vi "Delete_unwanted_rows.vi"(1 "Selected Rows":i32[](array[numeric]), 2 "Filename":path) -> ()   [LabVIEW 2015]
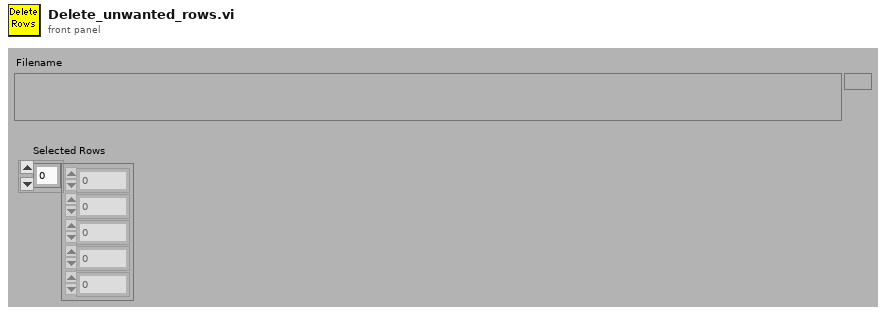
[diagram p1: front panel]
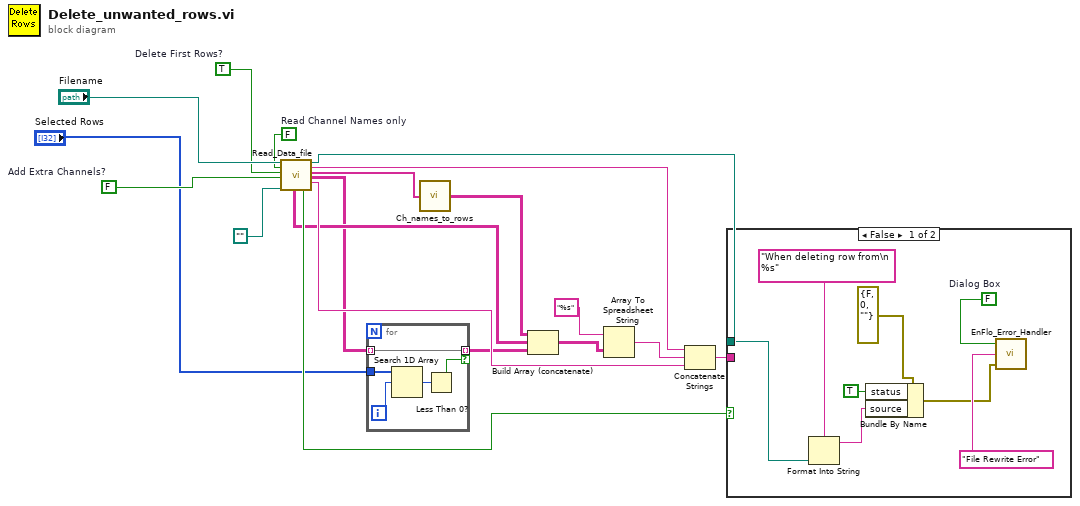
[diagram p0: block diagram]
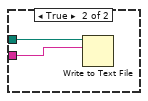
[diagram p2: hidden frame]
diagram:
  w1 = TRUE  # Delete First Rows?
  w5 = FALSE  # Add Extra Channels?
  w17 = FALSE  # Read Channel Names only
  n1 = call "Read_Data_file.vi"("Results file"="Filename", "Read Channel Names only"=w17, "Delete First Rows?"=w1, "Add Extra Channels?"=w5, "Template File"=path "") -> ("Deleted Rows"=w6:string[][], "EOF?"=w7:bool, "Results file Out"=w8:path, "String Before"=w15:string, "Ch names Out"=w14:string[], "Channel Values Out"=w3:string[][], "String After"=w10:string)  [unwired: 1 in, 7 out]
  n2 = for {
    tunnel: "Selected Rows" -> [w24]
    tunnel: w3 -> [w21] mode=indexing
    tunnel: [w21] -> w2 mode=indexing if=w20
    i -> [w23]
    n3 = Search 1D Array(1D array=w24, element=w23) -> (index of element=w22:i32)  [unwired: 1 in]
    n4 = Less Than 0?(x=w22) -> (x < 0?=w20:bool)
  }
  n5 = call "Ch_names_to_rows.vi"("Channel Names"=w14) -> ("3 Row names"=w13:string[][])
  n6 = Build Array (concatenate)(w13, w6, w2) -> (w12:string[][])
  n7 = Array To Spreadsheet String(array=w12, 3:"%s" ("format string")) -> (spreadsheet string=w11:string)  [unwired: 1 in]
  n8 = Concatenate Strings(w15, w11, w10) -> (w9:string)
  n9 = case shown="False" w7 {
    tunnel: w9 -> [_ w34]
    tunnel: w8 -> [w27 w33]
    frame False {
      w32 = FALSE  # Dialog Box
      n10 = Format Into String(format string="When deleting row from\n  %s", w27) -> (resulting string=w26:string)  [unwired: 2 in, 1 out]
      n11 = Bundle By Name(cluster=errorcluster {"status"=FALSE, "code"=0, "source"=""} ("error in (no error)"), "status"=TRUE, "source"=w26) -> (w29:errorcluster)
      n12 = call "EnFlo_Error_Handler.vi"("error in (no error)"=w29, "Error Type"="File Rewrite Error", "Dialog Box (T)"=w32) -> ()  [unwired: 3 out]
    }
    frame True {
      n13 = Write to Text File(file (use dialog)=w33, text=w34) -> ()  [unwired: 2 in, 3 out]
    }
  }
